vi "注册账号.vi"() -> ()   [LabVIEW 2018]
panel:
  in  "确定按钮":bool
  out "当前时间":timestamp
  out "字符串":string
  in  "密码":path=path "E:/登陆系统重写/密码.txt"
  in  "账号":path=path "E:/登陆系统重写/账户.txt"
  in  "验证码":string
  in  "重复密码":string
  in  "密码":string
  in  "账号":string
  # "注册账号"
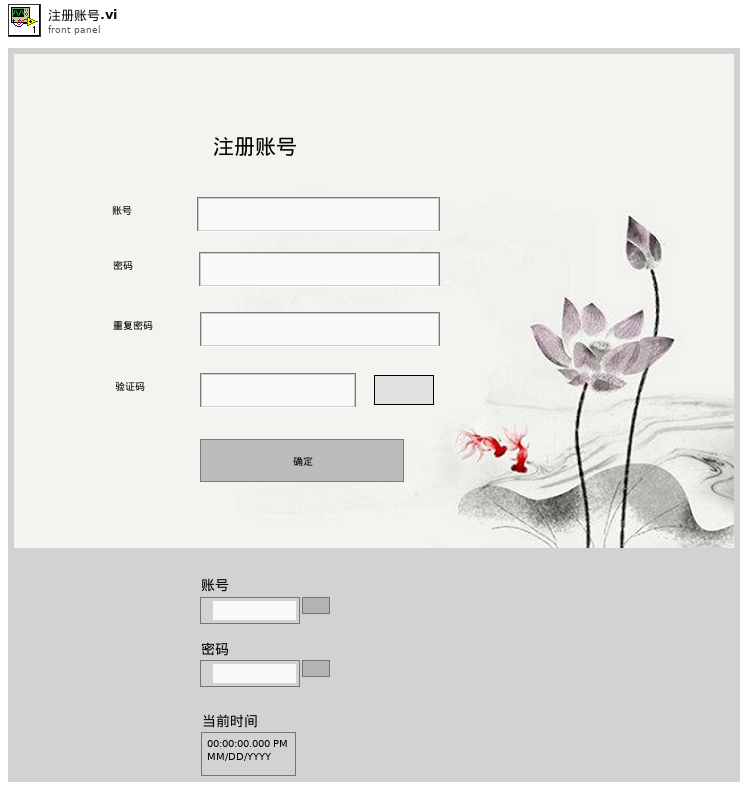
[diagram p1: front panel]
types:
  T1 = enum16{"open", "replace", "create", "open or create", "replace or create", "replace or create with confirmation"}
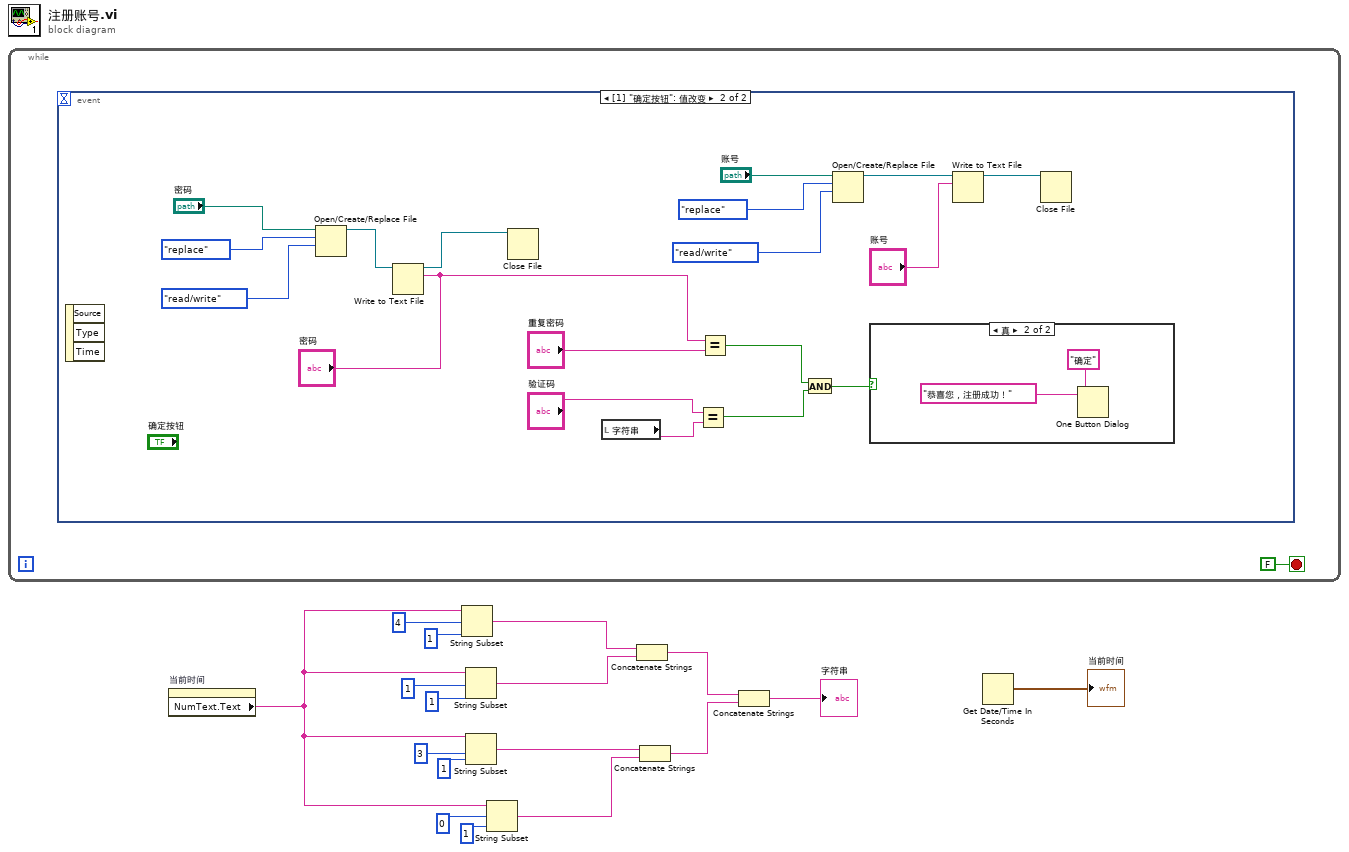
[diagram p0: block diagram]
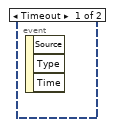
[diagram p2: hidden frame]
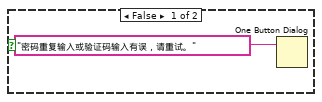
[diagram p3: hidden frame]
diagram:
  n1 = while {
    stop <- FALSE stop-if-true
    n2 = event shown="[1] \"确定按钮\": 值改变" {
      selector: _ -> [_ _]
      dyn-events: _ -> [_ _]
      timeout: _ -> [_ _]
      event Timeout {
        n3 = event-data() -> ()  [unwired: 1 in, 3 out]
      }
      event "确定按钮": Value Change {
        n4 = event-data() -> ()  [unwired: 1 in, 3 out]
        n5 = Open/Create/Replace File(file path (use dialog)="密码", operation (0:open)=T1."replace" ("操作(0:open)"), access (0:read/write)=enum16{"read/write", "read-only", "write-only"}."read/write" ("权限(0:read/write)")) -> (refnum out=w25:refnum<file>)  [unwired: 3 in, 2 out]
        n6 = Write to Text File(file (use dialog)=w25, text="密码") -> (refnum out=w26:refnum<file>)  [unwired: 2 in, 2 out]
        n7 = Close File(refnum=w26) -> ()  [unwired: 1 in, 2 out]
        n8 = local read "字符串"() -> (w20:string)
        n9 = Equal?(x="验证码", y=w20) -> (x = y?=w19:bool)
        n10 = Equal?(x="密码", y="重复密码") -> (x = y?=w22:bool)
        n11 = And(x=w22, y=w19) -> (x .and. y?=w30:bool)
        n12 = Open/Create/Replace File(file path (use dialog)="账号", operation (0:open)=T1."replace" ("操作(0:open)"), access (0:read/write)=enum16{"read/write", "read-only", "write-only"}."read/write" ("权限(0:read/write)")) -> (refnum out=w36:refnum<file>)  [unwired: 3 in, 2 out]
        n13 = case shown="真" w30 {
          frame False {
            n14 = One Button Dialog(message="密码重复输入或验证码输入有误，请重试。" ("消息")) -> ()  [unwired: 1 in, 1 out]
          }
          frame True {
            n15 = One Button Dialog(message="恭喜您，注册成功！" ("消息"), button name ("OK")="确定" ("按钮名称（“确定”）")) -> ()  [unwired: 1 out]
          }
        }
        n16 = Write to Text File(file (use dialog)=w36, text="账号") -> (refnum out=w35:refnum<file>)  [unwired: 2 in, 2 out]
        n17 = Close File(refnum=w35) -> ()  [unwired: 1 in, 2 out]
      }
    }
  }
  n18 = property on="当前时间" class="AbsTime (严格)"() -> ("NumText.Text"=w13:string)  [unwired: 2 in, 2 out]
  n19 = String Subset(string=w13, offset (0)=4 ("偏移量(0)"), length (rest)=1 ("长度（剩余）")) -> (substring=w17:string)
  n20 = String Subset(string=w13, offset (0)=1 ("偏移量(0)"), length (rest)=1 ("长度（剩余）")) -> (substring=w16:string)
  n21 = String Subset(string=w13, offset (0)=3 ("偏移量(0)"), length (rest)=1 ("长度（剩余）")) -> (substring=w15:string)
  n22 = String Subset(string=w13, offset (0)=0 ("偏移量(0)"), length (rest)=1 ("长度（剩余）")) -> (substring=w14:string)
  n23 = Concatenate Strings(w17, w16) -> (w12:string)
  n24 = Concatenate Strings(w15, w14) -> (w11:string)
  n25 = Concatenate Strings(w12, w11) -> (→"字符串":string)
  n26 = Get Date/Time In Seconds() -> (seconds since 1Jan1904=→"当前时间":timestamp)
